vi "Set_Frames.vi"(8 "error in (no error)":errorcluster, 10 "Frames":i32, 11 "Avantes in":refnum<class "Avantes.lvclass">) -> (0 "error out":errorcluster, 3 "Avantes out":refnum<class "Avantes.lvclass">)   [LabVIEW 2020, in "Avantes.lvclass"]
uses:
  <instrlib>/Classes/CCD/Avantes/Avantes.lvclass
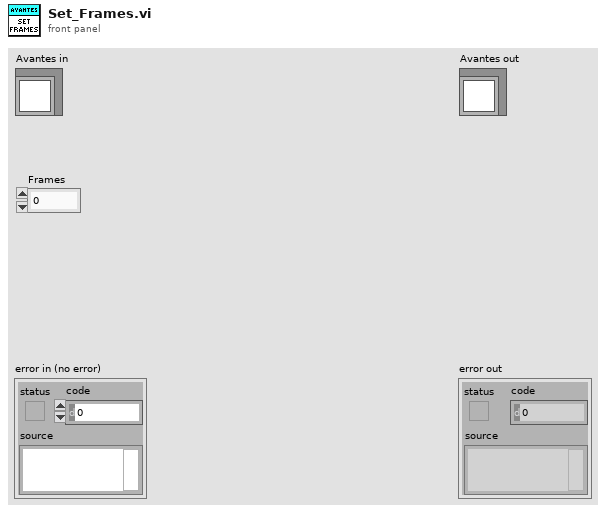
[diagram p1: front panel]
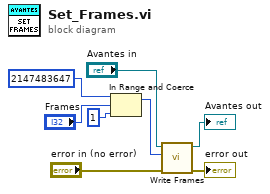
[diagram p0: block diagram]
diagram:
  n1 = In Range and Coerce(upper limit=2147483647, x="Frames", lower limit=1) -> (coerced(x)=w2:i32)  [unwired: 1 out]
  n2 = call-dynamic "Write Frames.vi"("error in (no error)"="error in (no error)", "Frames"=w2, "Avantes in"="Avantes in") -> ("error out"=→"error out":errorcluster, "Avantes out"=→"Avantes out":refnum<class "Avantes.lvclass">)  [unwired: 7 in]
